vi "WMS_Query.vi"(0 "System no.":i32=1 min=1 max=4 step=1, 2 "Axes to query":string[](array[string]), 3 "All axes?":bool, 4 "Axis identifier?":bool=TRUE, 5 "error in":errorcluster) -> (14 "Wave storage max.":dbl[](array[numeric]), 19 "error out":errorcluster)   [LabVIEW 2020]
doc: "Returns maximum size of wave-point storage for specified axes.\n\nC-886: Axes to query are identical with wave table numbers, which can be 1 to100. All axes? must be FALSE.\n\nC-887: Axes to query are identical with wave table numbers, which can be 1 to100. All axes? must be FALSE. \n\nE-517, E-518: Axes to query are identical with wave table numbers, which can be 1 to 3. All axes must be FALSE. \n\nE-710: If All axes = TRUE, then Axis identifier must be TRUE\n\nE-761: All axes must be FALSE. Axis to query is identical with wave table number, which can be 1 to 4."
panel:
  # "Returns maximum size of wave-point storage for specified axes."
  # "If all axes: use"
  # "Query"
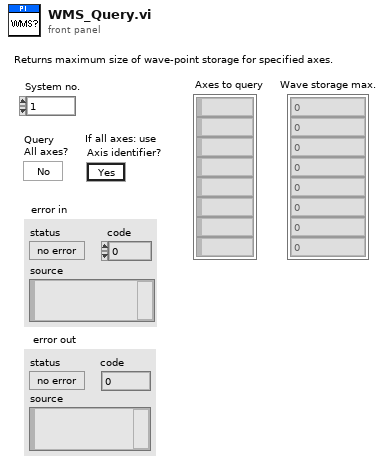
[diagram p1: front panel]
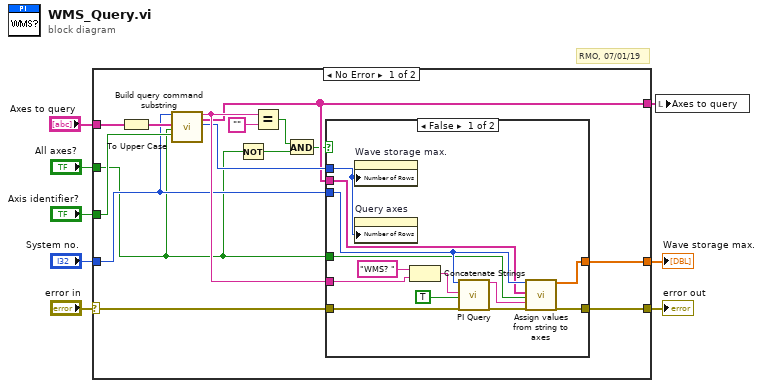
[diagram p0: block diagram]
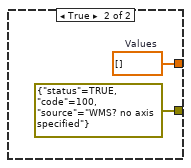
[diagram p2: hidden frame]
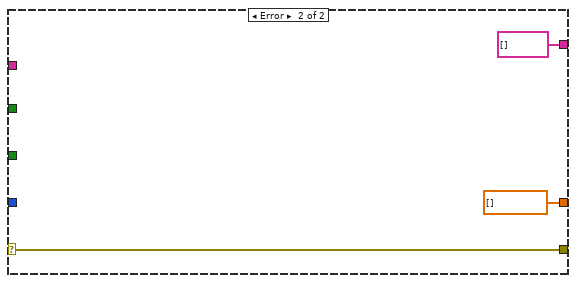
[diagram p3: hidden frame]
diagram:
  # "RMO, 07/01/19"
  n1 = case shown="No Error" "error in" {
    selector: "error in" -> [w11 w39]
    tunnel: [w23 dbl[] [] ("Values")] -> w8
    tunnel: "Axes to query" -> [w22 _]
    tunnel: [w10 w39] -> w6
    tunnel: "Axis identifier?" -> [w19 _]
    tunnel: "System no." -> [w16 _]
    tunnel: [w15 string[] [] ("Axes to query out")] -> w3
    tunnel: "All axes?" -> [w14 _]
    frame No Error {
      n2 = To Upper Case(1:w22) -> (0:w20:string[])
      n3 = call "Build query command substring.vi"("System no."=w16, "Axes to query in"=w20, "Query\nAll axes?"=w14, "For all axes: use\nAxis identifier?"=w19) -> ("Command substring"=w18:string, "Axes to query out"=w15:string[], "Number of rows"=w17:u32)  [unwired: 2 in, 11 out]
      n4 = Not(x=w14) -> (.not. x?=w12:bool)
      n5 = Equal?(x=w18, y="" ("x")) -> (x = y?=w13:bool)
      n6 = And(x=w13, y=w12) -> (x .and. y?=w9:bool)
      n7 = case shown="False" w9 {
        tunnel: [w33 w37] -> w23
        tunnel: w18 -> [w32 _]
        tunnel: w17 -> [w31 _]
        tunnel: w16 -> [w30 _]
        tunnel: w15 -> [w29 _]
        tunnel: w14 -> [w28 _]
        tunnel: w11 -> [w27 _]
        tunnel: [w26 errorcluster {"status"=TRUE, "code"=100, "source"="WMS? no axis specified"} ("error out")] -> w10
        frame False {
          n8 = property on="Wave storage max." class="Arr (strict)"("Number of Rows"=w31) -> ()  [unwired: 2 in, 2 out]
          n9 = property on="Query axes" class="Arr (strict)"("Number of Rows"=w31) -> ()  [unwired: 2 in, 2 out]
          n10 = Concatenate Strings("WMS? ", w32) -> (w34:string)
          n11 = call "PI Query.vi"("System no."=w30, "String to send"=w34, "Attach termination char.?"=TRUE ("Attach Linefeed?"), "error in"=w27) -> ("String read"=w24:string, "error out"=w25:errorcluster)  [unwired: 3 in, 11 out]
          n12 = call "Assign values from string to axes.vi"("System no."=w30, "Queried axes"=w29, "All axes queried?"=w28, "Input String"=w24, "error in"=w25) -> ("Values"=w33:dbl[], "error out"=w26:errorcluster)  [unwired: 4 in, 9 out]
        }
        frame True {
          w37 = dbl[] []  # Values
        }
      }
    }
    frame Error {
    }
  }
  "error out" <- w6
  "Wave storage max." <- w8
  n13 = local write "Axes to query"(w3) -> ()
